vi "testMultiDimensionalArray.vi"(8 "error in (no error)":errorcluster, 11 "TestCase in":refnum<class "EasyXMLTest.lvclass">) -> (0 "error out":errorcluster, 3 "TestCase out":refnum<class "EasyXMLTest.lvclass">)   [LabVIEW 2013, in "EasyXMLTest.lvclass"]
doc: "Verify that error in is not overwritten"
uses:
  EasyXMLTest.lvclass
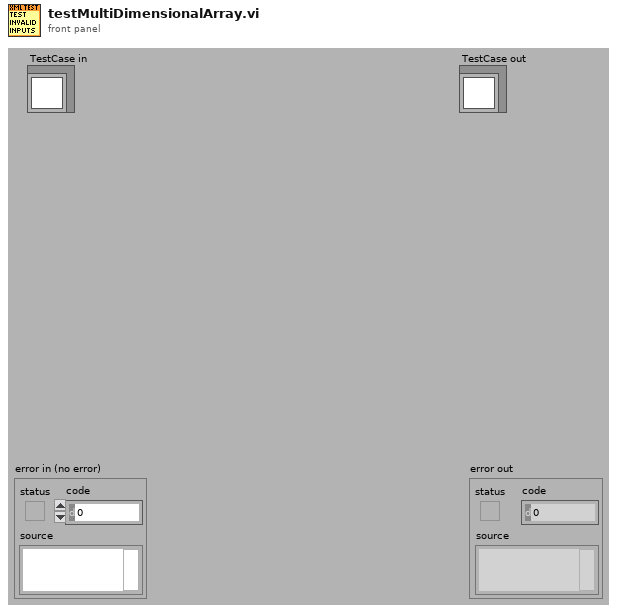
[diagram p1: front panel]
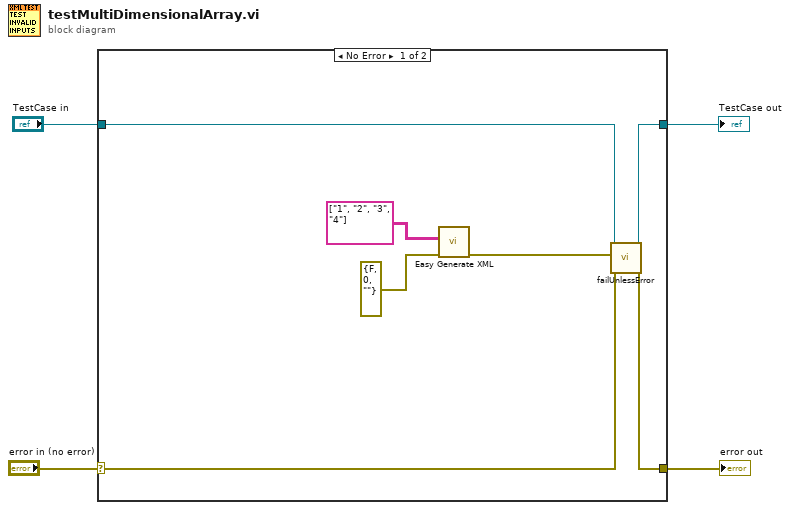
[diagram p0: block diagram]
diagram:
  n1 = case shown="No Error" "error in (no error)" {
    selector: "error in (no error)" -> [w8 w13]
    tunnel: [w7 w13] -> w2
    tunnel: [w11 w12] -> w1
    tunnel: "TestCase in" -> [w9 w12]
    frame No Error {
      n2 = call "Easy Generate XML.vi"("error in (no error)"=errorcluster {"status"=FALSE, "code"=0, "source"=""}, "LabVIEW Data"=string[][] [["1", "2"], ["3", "4"]]) -> ("error out"=w10:errorcluster)  [unwired: 8 in, 1 out]
      n3 = call-dynamic "failUnlessError.vi"("error in (no error)"=w8, "error"=w10, "TestCase in"=w9) -> ("error out"=w7:errorcluster, "TestCase out"=w11:refnum<class "EasyXMLTest.lvclass">)  [unwired: 7 in]
    }
    frame Error {
    }
  }
  "error out" <- w2
  "TestCase out" <- w1
